vi "test_udp_discovery_server.vi"() -> ()   [LabVIEW 2019]
uses:
  <vilib>/userDefined/High Color/IMAQdx.ctl
  <vilib>/vision/driver/NI_Vision_Acquisition_Software.lvlib
panel:
  out "Image Pixels (U16)":u16[][](array[numeric])
  out "Image Pixels (I16)":i16[][](array[numeric])
  out "error out 2":errorcluster
  out "Image Pixels (U8)":u8[][](array[numeric])
  in  "Optional Rectangle":i32[](array[numeric])=[98, 180, 115, 197]
  out "error out":errorcluster
  out "Image":T1(plugin-control)
  in  "정지":bool
  in  "Session In":T2
  out "Client IP Address":string
  in  "stop":bool
  out "n":i32
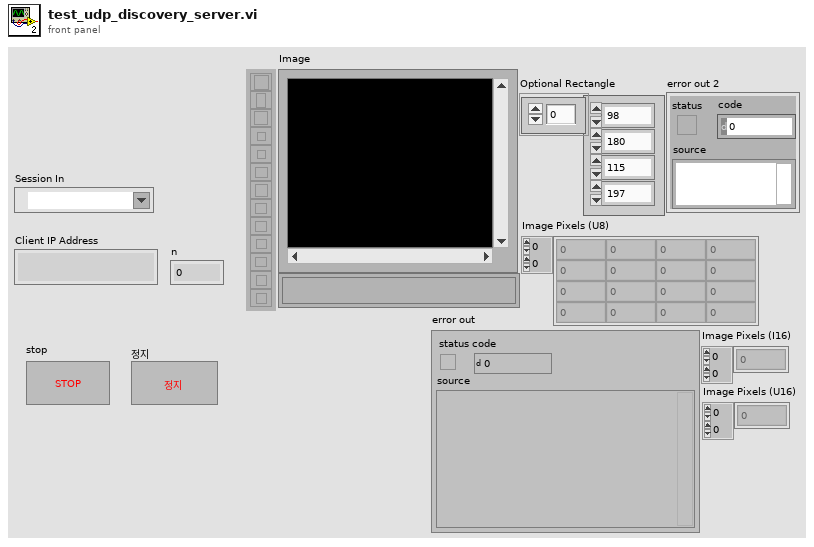
[diagram p1: front panel]
types:
  T1 = typedef "IMAQ Image.ctl" = refnum<image>
  T2 = typedef "IMAQdx.ctl" = refnum<k21>
  T3 = typedef "Image Type" = u32
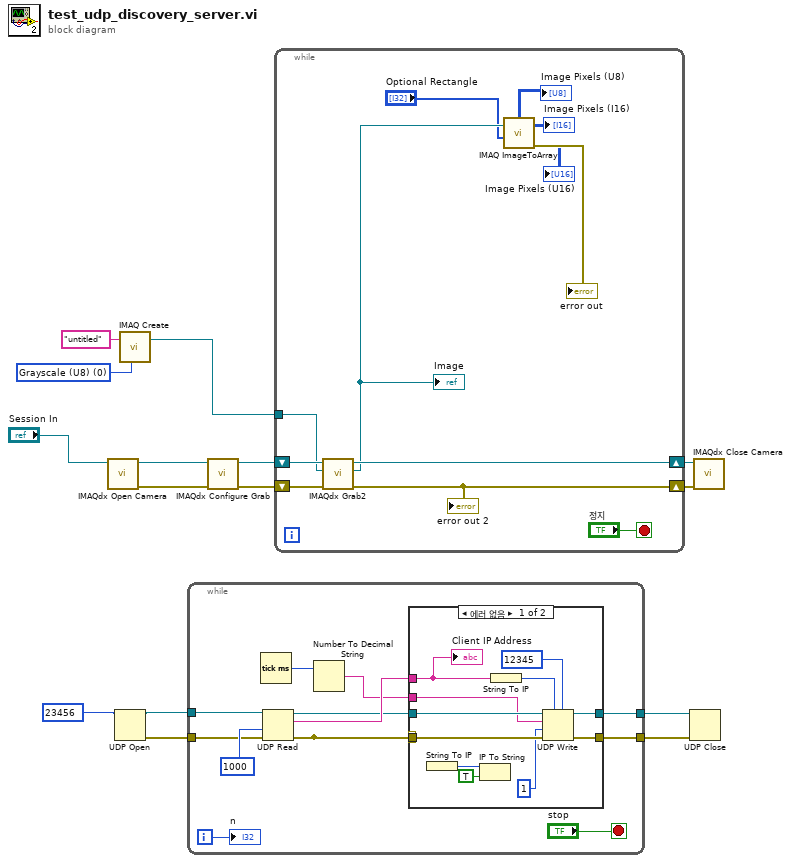
[diagram p0: block diagram]
diagram:
  w1 = T3 0 items=["Grayscale (U8)", "Grayscale (I16)", "Grayscale (SGL)", "Complex (CSG)", "RGB (U32)", "HSL (U32)", "RGB (U64)", "Grayscale (U16)"] ("Image Type")
  n1 = call <vilib>:"IMAQdx Open Camera.vi"("Session In"="Session In") -> ("error out"=w10:errorcluster, "Session Out"=w9:T2)  [unwired: 9 in]
  n2 = UDP Open(11:u16 23456 ("port")) -> (port=w15:refnum<k16>, 0:w14:errorcluster)  [unwired: 4 in, 1 out]
  n3 = call "IMAQ Create"("Image Name"="untitled", "Image Type"=w1) -> ("New Image"=w2:T1)  [unwired: 3 in, 1 out]
  n4 = while {
    tunnel: w15 -> [w26]
    tunnel: w14 -> [w25]
    tunnel: [w20] -> w12
    tunnel: [w19] -> w11
    i -> [w18]
    stop <- "stop" stop-if-true
    n5 = Tick Count (ms)() -> (millisecond timer value=w17:u32)
    n6 = UDP Read(connection ID=w26, timeout ms (25000)=1000, 8:w25) -> (data out=w24:string, error out=w22:errorcluster, 3:w23:refnum<k16>)  [unwired: 1 in, 2 out]
    n7 = Number To Decimal String(number=w17) -> (decimal integer string=w16:string)  [unwired: 1 in]
    n8 = case shown="에러 없음" w22 {
      selector: w22 -> [w33 _]
      tunnel: w24 -> [w30 _]
      tunnel: w23 -> [w34 w39]
      tunnel: w22 -> [_ _]
      tunnel: [w32 w39] -> w20
      tunnel: [w31 _] -> w19
      tunnel: w16 -> [w28 _]
      frame No Error {
        n9 = String To IP() -> (0:w37:u32)  [unwired: 1 in]
        n10 = IP To String(1:TRUE ("dot notation? (F)"), 2:w37) -> ()  [unwired: 1 out]
        n11 = String To IP(1:w30) -> (0:w35:u32)
        n12 = UDP Write(address=w35, port or service name=u16 12345 ("port"), connection ID=w34, data in=w28, 8:w33, 9:1 ("타임아웃 ms (25000)")) -> (error out=w31:errorcluster, 3:w32:refnum<k16>)
        "Client IP Address" <- w30
      }
      frame Error {
      }
    }
    "n" <- w18
  }
  n13 = call <vilib>:"IMAQdx Configure Grab.vi"("error in"=w10, "Session In"=w9) -> ("error out"=w7:errorcluster, "Session Out"=w8:T2)  [unwired: 8 in]
  n14 = while {
    shift-right: [w49] -> w5
    shift-left: w8 -> [w51]
    shift-right: [w46] -> w6
    shift-left: w7 -> [w50]
    tunnel: w2 -> [w47]
    stop <- "정지" stop-if-true
    n15 = call <vilib>:"IMAQdx Grab2.vi"("error in"=w50, "Image In"=w47, "Session In"=w51) -> ("error out"=w46:errorcluster, "Image Out"=w45:T1, "Session Out"=w49:T2)  [unwired: 5 in, 1 out]
    "Image" <- w45
    "error out 2" <- w46
    n16 = call "IMAQ ImageToArray"("Optional Rectangle"="Optional Rectangle", "Image"=w45) -> ("Image Pixels (U16)"=→"Image Pixels (U16)":u16[][], "error out"=→"error out":errorcluster, "Image Pixels (U8)"=→"Image Pixels (U8)":u8[][], "Image Pixels (I16)"=→"Image Pixels (I16)":i16[][])  [unwired: 2 in, 1 out]
  }
  n17 = UDP Close(connection ID=w12, 8:w11) -> ()  [unwired: 2 out]
  n18 = call <vilib>:"IMAQdx Close Camera.vi"("error in"=w6, "Session In"=w5) -> ()  [unwired: 9 in, 1 out]
